vi "Set Parameter.vi"(8 "error in (no error)":errorcluster, 10 "Parameter in":refnum<class "AbstractData.lvclass">, 11 "Simulated ParameterDevice in":refnum<class "Simulated ParameterDevice.lvclass">) -> (0 "error out":errorcluster, 3 "Simulated ParameterDevice out":refnum<class "Simulated ParameterDevice.lvclass">)   [LabVIEW 2014, in "Simulated ParameterDevice.lvclass"]
uses:
  Simulated ParameterDevice.lvclass
  Framework/Model/Data/AbstractData/AbstractData.lvclass
  Framework/Model/Data/DataSingleElement/DataSingleElement.lvclass
  Simulated ParameterDevice.lvclass/Simulated ParameterDevice.ctl
  Framework/Interfaces/Observable Actor/Observable Actor.lvclass
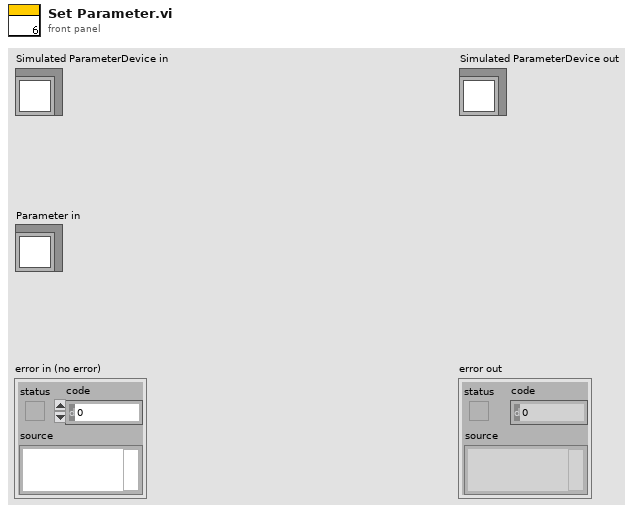
[diagram p1: front panel]
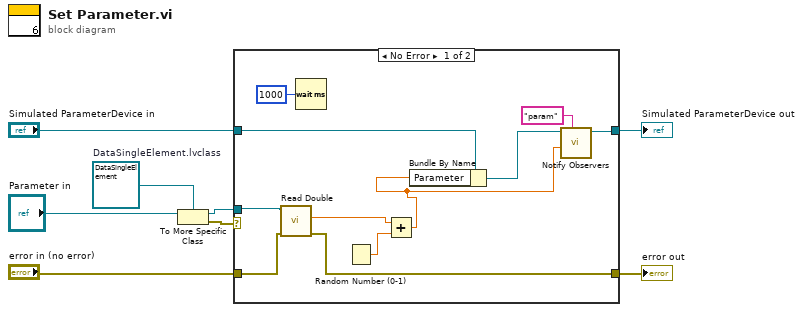
[diagram p0: block diagram]
diagram:
  w1 = refnum<class "DataSingleElement.lvclass"> refnum  # DataSingleElement.lvclass
  n1 = To More Specific Class(target class=w1, reference="Parameter in") -> (specific class reference=w7:refnum<class "DataSingleElement.lvclass">, error out=w8:errorcluster)  [unwired: 1 in]
  n2 = case shown="No Error" w8 {
    tunnel: w7 -> [w14 _]
    tunnel: "Simulated ParameterDevice in" -> [w19 w21]
    tunnel: "error in (no error)" -> [w13 w20]
    tunnel: [w12 w20] -> w4
    tunnel: [w17 w21] -> w3
    frame No Error {
      n3 = call "Read Double.vi"("error in (no error)"=w13, "DataSingleElement in"=w14) -> ("error out"=w12:errorcluster, "value"=w10:dbl)  [unwired: 7 in, 1 out]
      n4 = Wait (ms)(milliseconds to wait=u32 1000) -> ()  [unwired: 1 out]
      n5 = Random Number (0-1)() -> (number: 0 to 1=w11:dbl)
      n6 = Add(x=w10, y=w11) -> (x+y=w9:dbl)
      n7 = Bundle By Name(cluster=w19, "Parameter"=w9) -> (w18:refnum<class "Simulated ParameterDevice.lvclass">)
      n8 = call "Notify Observers.vi"("name"="param", "value"=w9, "Observable Actor in"=w18) -> ("Observable Actor out"=w17:refnum<class "Simulated ParameterDevice.lvclass">)  [unwired: 7 in, 1 out]
    }
    frame Error {
    }
  }
  "error out" <- w4
  "Simulated ParameterDevice out" <- w3
